vi "Is Status Null.vi"(8 "error in (no error)":errorcluster, 11 "status pointer in":refnum<class "Status.lvclass">) -> (0 "error out":errorcluster, 2 "null?":bool, 3 "status pointer out":refnum<class "Status.lvclass">)   [LabVIEW 2017, in "DSF Core.lvlib" / "Status.lvclass"]
uses:
  Status.lvclass
  C:/Git/DSF/LabVIEW-Memory/Source/Classes/Pointer/Pointer.lvclass
  LabVIEW-Memory/Source/Classes/Pointer/Pointer.lvclass
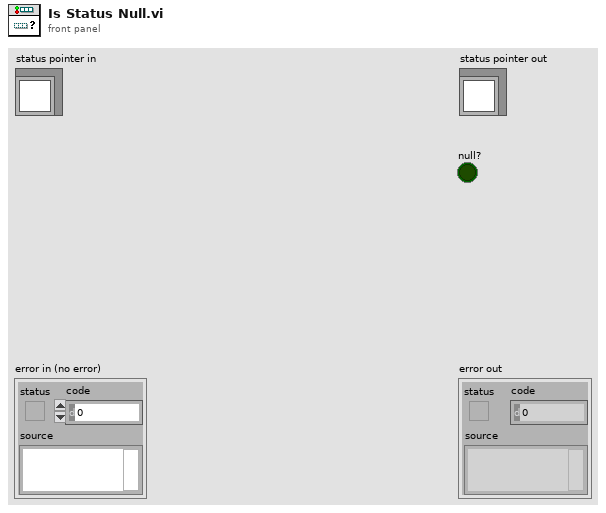
[diagram p1: front panel]
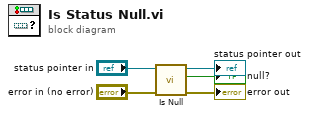
[diagram p0: block diagram]
diagram:
  n1 = call "Is Null.vi"("error in (no error)"="error in (no error)", "Pointer in"="status pointer in") -> ("error out"=→"error out":errorcluster, "null?"=→"null?":bool, "Pointer out"=→"status pointer out":refnum<class "Status.lvclass">)  [unwired: 7 in]
